vi "ax+b.vi"(1 "x":i32, 2 "b":i32, 3 "a":i32) -> (0 "y":i32)   [LabVIEW 2012]
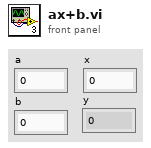
[diagram p1: front panel]
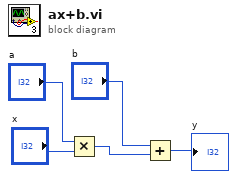
[diagram p0: block diagram]
diagram:
  n1 = Multiply(x="a", y="x") -> (x*y=w3:i32)
  n2 = Add(x="b", y=w3) -> (x+y=→"y":i32)
